vi "CTRE_Phoenix_MotorControl_BufferedTrajectoryPointStream_SetDeviceReference.vi"(8 "error in (no error)":errorcluster, 9 "Test Mode Only":bool, 10 "refnum name":string="My TrajPointStream RefNum", 11 "BufferedTrajectoryPointStream_DevRef":T1) -> (0 "error out":errorcluster, 3 "BufferedTrajectoryPointStream_DevRef":T1)   [LabVIEW 2019]
uses:
  <vilib>/Rock Robotics/WPI/ThirdParty/Phoenix-LabVIEW/Motor Controller/Controls/CTRE_Phoenix_MotorControl_BufferedTrajectoryPointStream_DeviceRef.ctl
  <vilib>/Rock Robotics/WPI/Utilities/Refnum Registry Operation.ctl
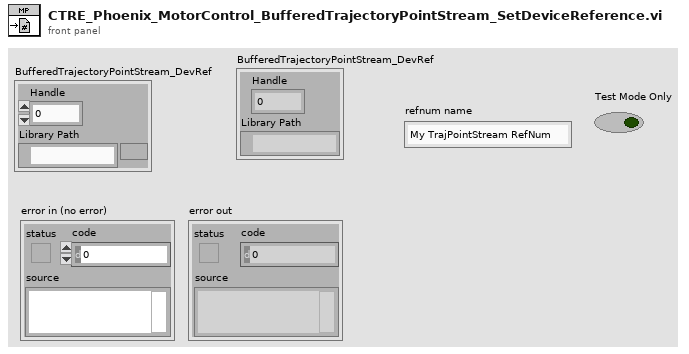
[diagram p1: front panel]
types:
  T1 = typedef "CTRE_Phoenix_MotorControl_BufferedTrajectoryPointStream_DeviceRef.ctl" = cluster{"Handle":u64, "Library Path":path}
  T2 = typedef "Refnum Registry Operation.ctl" = enum16{"set", "get", "delete", "get all names", "read name"}
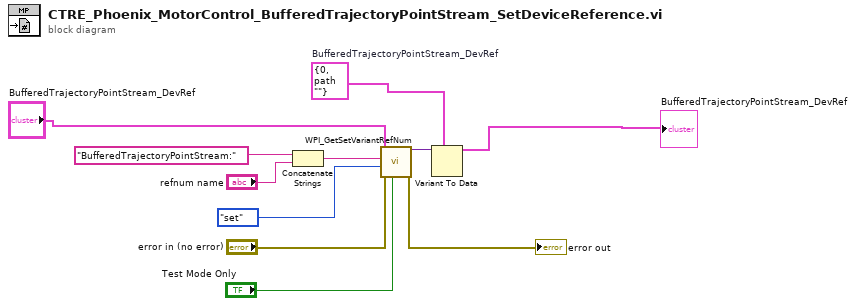
[diagram p0: block diagram]
diagram:
  w3 = T1 {"Handle"=0, "Library Path"=path ""}  # BufferedTrajectoryPointStream_DevRef
  n1 = Concatenate Strings("BufferedTrajectoryPointStream:", "refnum name") -> (w11:string)
  n2 = call <vilib>:"WPI_GetSetVariantRefNum.vi"("Test Mode Only"="Test Mode Only", "error in (no error)"="error in (no error)", "Operation"=Refnum_Registry_Operation."set" ("menu"), "refnum name"=w11, "DevRef"="BufferedTrajectoryPointStream_DevRef") -> ("error out"=→"error out":errorcluster, "DevRef"=w9:variant)  [unwired: 4 in, 1 out]
  n3 = Variant To Data(type=w3, Variant=w9) -> (data=→"BufferedTrajectoryPointStream_DevRef":T1)  [unwired: 1 in, 1 out]
